vi "write_params.vi"(8 "error in (no error)":errorcluster, 10 "params":T1={"n_components"=2.0, "affinity"="nearest_neighbors", "gamma"={"gamma_type"="None", "gamma_float"=0.0}, "random_state"=0.0, "eigen_solver"="arpack", "n_neighbors"={"n_neighbors_type"="None", "n_neighbors_int"=0.0}, "n_jobs"=0.0}, 11 "SpectralEmbedding in":refnum<class "SpectralEmbedding.lvclass">) -> (0 "error out":errorcluster, 3 "SpectralEmbedding out":refnum<class "SpectralEmbedding.lvclass">)   [LabVIEW 2020, in "SpectralEmbedding.lvclass"]
uses:
  SpectralEmbedding.lvclass
  Controls/spectral_embedding_params.ctl
  SpectralEmbedding.lvclass/SpectralEmbedding.ctl
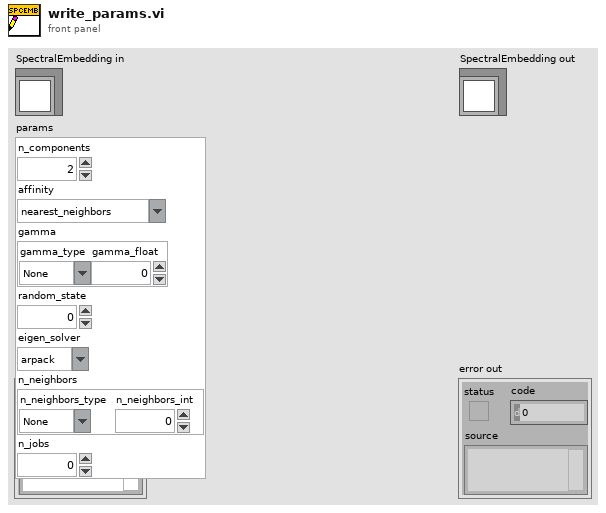
[diagram p1: front panel]
types:
  T1 = typedef "spectral_embedding_params.ctl" = cluster{"n_components":dbl, "affinity":string, "gamma":cluster{"gamma_type":string, "gamma_float":dbl}, "random_state":dbl, "eigen_solver":string, "n_neighbors":cluster{"n_neighbors_type":string, "n_neighbors_int":dbl}, "n_jobs":dbl}
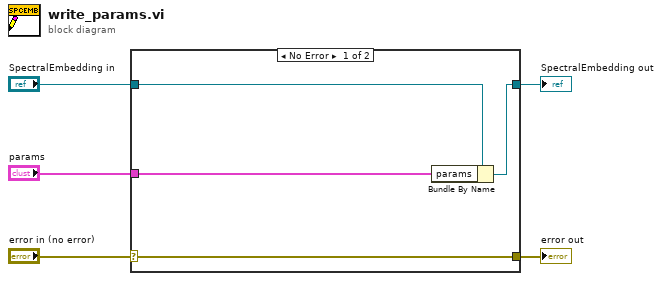
[diagram p0: block diagram]
diagram:
  n1 = case shown="No Error" "error in (no error)" {
    selector: "error in (no error)" -> [w9 w10]
    tunnel: [w9 w10] -> w4
    tunnel: [w7 w11] -> w2
    tunnel: "SpectralEmbedding in" -> [w8 w11]
    tunnel: "params" -> [w6 _]
    frame No Error {
      n2 = Bundle By Name(cluster=w8, "params"=w6) -> (w7:refnum<class "SpectralEmbedding.lvclass">)
    }
    frame Error {
    }
  }
  "error out" <- w4
  "SpectralEmbedding out" <- w2
